vi "Get CPMG Params.vi"(11 "CPMG Parameters":T1={"Path to CPMG Burner"=path "C:/Users/Loncar/Desktop/ESR VIs - Srujan/Sam Kim/PB/SpinEchoBurn.exe", "Window 1 time (s)"=3e-06, "Window 1 active channels"=[FALSE, FALSE, FALSE, TRUE], "Window 10 time (s)"=3e-06, "Window 10 active channels"=[FALSE, FALSE, FALSE, TRUE], "Window 2 time (s)"=0.0, "Window 2 active channels"=[], "Window 4 min time (s) "=0.0, "Window 4 active channels"=[FALSE], "Window 8 time (s)"=7.5e-07, "Window 8 active channels"=[FALSE, FALSE, FALSE, TRUE], "Window 9 time (s)"=2e-07, "Window 9 active channels "=[FALSE, FALSE, TRUE, TRUE], "# delay time points"=1, "Window 11 time (s)"=0.0, "Window 11 active channels"=[FALSE, FALSE, TRUE, TRUE], "Window 12 time (s)"=1e-07, "Window 12 active channels"=[], "Window 4 max time (s)"=0.0, "Window 3 time (s)"=0.0, "Window 5 time (s)"=5e-06, "Window 3 active channels"=[TRUE, FALSE, FALSE, FALSE], "Window 5 active channels"=[TRUE, FALSE, FALSE, FALSE], "# pi pulses"=1, "# samples before track"=0} {"# pi pulses" min=1; "# delay time points" min=2}) -> (0 "max time":dbl, 1 "min time":dbl, 2 "# time points":i32, 3 "# samples":i32, 4 "Window Params Args":string)   [LabVIEW 2012]
uses:
  Window Parameters-CPMG.ctl
panel:
  # "Green AOM"
  # "Initialization"
  # "All off"
  # "Wait"
  # "MW pulse 1\n(pi/2)"
  # "MW"
  # "Free precession\n(Tau/2)"
  # "All off"
  # "max: ~350"
  # "MW pulse 2\n(pi90)"
  # "MW90"
  # "Free precession (Tau/2)\nMW pulse 1 (pi/2)"
  # "Window 6 = Window 4\nWindow 7 = Window 3"
  # "All off\nMW"
  # "Green AOM"
  # "Wait for green"
  # "Green AOM,\ncounter clk"
  # "Readout"
  # "Green AOM"
  # "Repump"
  # "Green AOM,\ncounter clk"
  # "Reference"
  # "Wait (nominal)"
  # "All off"
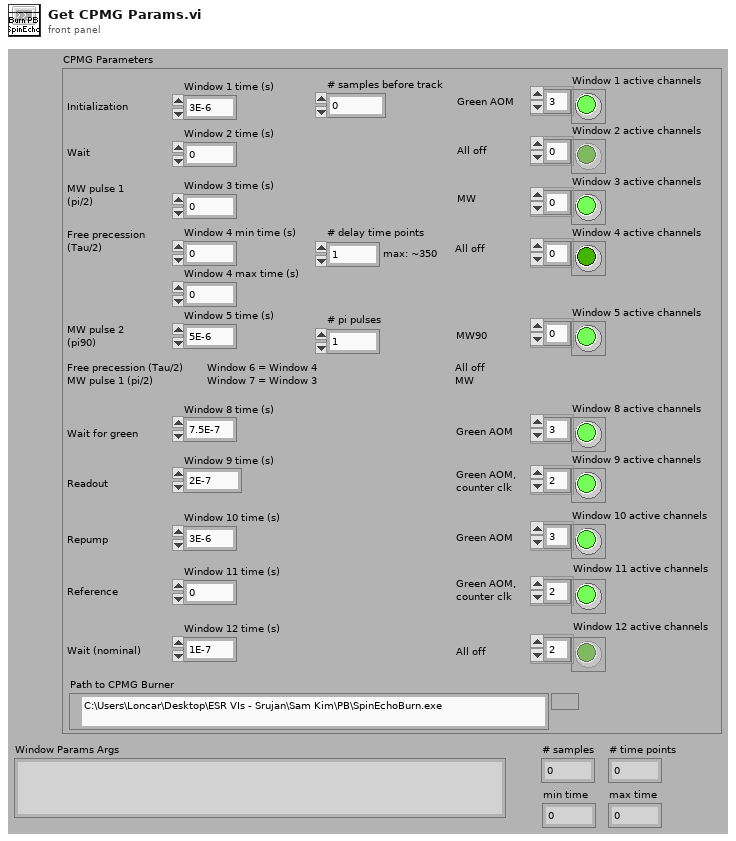
[diagram p1: front panel]
types:
  T1 = typedef "Window Parameters-CPMG.ctl" = cluster{"Path to CPMG Burner":path, "Window 1 time (s)":dbl, "Window 1 active channels":bool[], "Window 10 time (s)":dbl, "Window 10 active channels":bool[], "Window 2 time (s)":dbl, "Window 2 active channels":bool[], "Window 4 min time (s) ":dbl, "Window 4 active channels":bool[], "Window 8 time (s)":dbl, "Window 8 active channels":bool[], "Window 9 time (s)":dbl, "Window 9 active channels ":bool[], "# delay time points":i32, "Window 11 time (s)":dbl, "Window 11 active channels":bool[], "Window 12 time (s)":dbl, "Window 12 active channels":bool[], "Window 4 max time (s)":dbl, "Window 3 time (s)":dbl, "Window 5 time (s)":dbl, "Window 3 active channels":bool[], "Window 5 active channels":bool[], "# pi pulses":i32, "# samples before track":i32}
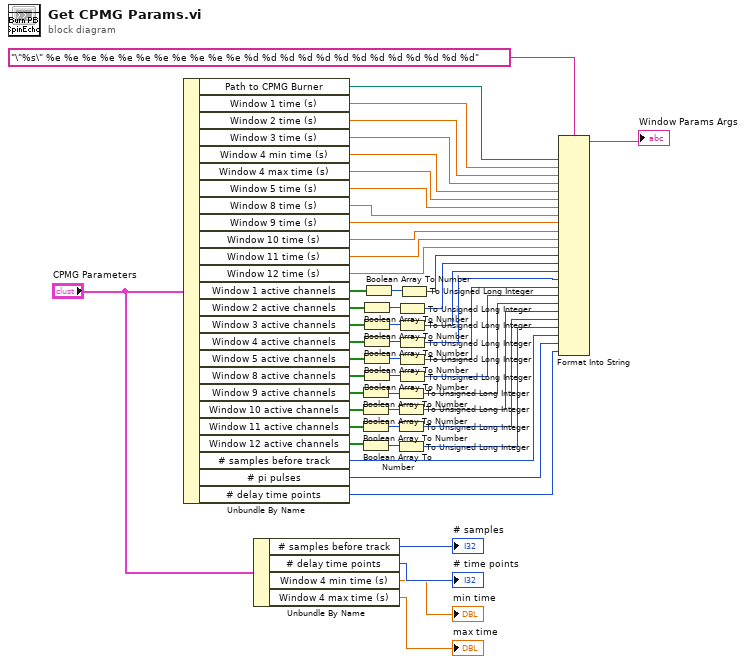
[diagram p0: block diagram]
diagram:
  n1 = Unbundle By Name("CPMG Parameters") -> ("Path to CPMG Burner"=w25:path, "Window 1 time (s)"=w24:dbl, "Window 2 time (s)"=w23:dbl, "Window 3 time (s)"=w22:dbl, "Window 4 min time (s)"=w21:dbl, "Window 4 max time (s)"=w20:dbl, "Window 5 time (s)"=w19:dbl, "Window 8 time (s)"=w18:dbl, "Window 9 time (s)"=w17:dbl, "Window 10 time (s)"=w16:dbl, "Window 11 time (s)"=w15:dbl, "Window 12 time (s)"=w14:dbl, "Window 1 active channels"=w7:bool[], "Window 2 active channels"=w6:bool[], "Window 3 active channels"=w13:bool[], "Window 4 active channels"=w5:bool[], "Window 5 active channels"=w4:bool[], "Window 8 active channels"=w12:bool[], "Window 9 active channels"=w11:bool[], "Window 10 active channels"=w10:bool[], "Window 11 active channels"=w9:bool[], "Window 12 active channels"=w8:bool[], "# samples before track"=w3:i32, "# pi pulses"=w2:i32, "# delay time points"=w1:i32)
  n2 = Unbundle By Name("CPMG Parameters") -> ("# samples before track"=→"# samples":i32, "# delay time points"=→"# time points":i32, "Window 4 min time (s)"=→"min time":dbl, "Window 4 max time (s)"=→"max time":dbl)
  n3 = Boolean Array To Number(Boolean array=w11) -> (number=w52:u32)
  n4 = Boolean Array To Number(Boolean array=w10) -> (number=w51:u32)
  n5 = Boolean Array To Number(Boolean array=w9) -> (number=w50:u32)
  n6 = Boolean Array To Number(Boolean array=w8) -> (number=w34:u32)
  n7 = Boolean Array To Number(Boolean array=w6) -> (number=w37:u32)
  n8 = Boolean Array To Number(Boolean array=w13) -> (number=w49:u32)
  n9 = Boolean Array To Number(Boolean array=w5) -> (number=w48:u32)
  n10 = Boolean Array To Number(Boolean array=w4) -> (number=w47:u32)
  n11 = Boolean Array To Number(Boolean array=w12) -> (number=w46:u32)
  n12 = Boolean Array To Number(Boolean array=w7) -> (number=w38:u32)
  n13 = To Unsigned Long Integer(number=w52) -> (unsigned 32bit integer=w41:u32)
  n14 = To Unsigned Long Integer(number=w51) -> (unsigned 32bit integer=w40:u32)
  n15 = To Unsigned Long Integer(number=w50) -> (unsigned 32bit integer=w39:u32)
  n16 = To Unsigned Long Integer(number=w34) -> (unsigned 32bit integer=w35:u32)
  n17 = To Unsigned Long Integer(number=w37) -> (unsigned 32bit integer=w36:u32)
  n18 = To Unsigned Long Integer(number=w49) -> (unsigned 32bit integer=w45:u32)
  n19 = To Unsigned Long Integer(number=w48) -> (unsigned 32bit integer=w44:u32)
  n20 = To Unsigned Long Integer(number=w47) -> (unsigned 32bit integer=w43:u32)
  n21 = To Unsigned Long Integer(number=w46) -> (unsigned 32bit integer=w42:u32)
  n22 = To Unsigned Long Integer(number=w38) -> (unsigned 32bit integer=w27:u32)
  n23 = Format Into String(format string="\"%s\" %e %e %e %e %e %e %e %e %e %e %e %d %d %d %d %d %d %d %d %d %d %d %d %d", w25, w24, w23, w22, w21, w20, w19, w18, w17, w16, w15, w14, w27, w36, w45, w44, w43, w42, w41, w40, w39, w35, w3, w2, w1) -> (resulting string=→"Window Params Args":string)  [unwired: 2 in, 1 out]
